vi "main_queque_manager.vi"(8 "error in":errorcluster, 9 "State insert position":T1, 10 "New states array":T2[](array[typedef]), 11 "Main state queue in":refnum<queue>) -> (0 "error out":errorcluster, 3 "Main state queue out":refnum<queue>)   [LabVIEW 2011, in "Fiberscope_library.lvlib"]
uses:
  Fiberscope_library.lvlib
  typedefs/main_state_cluster.ctl
  typedefs/main_state_enum.ctl
  typedefs/state_insert_position_enum.ctl
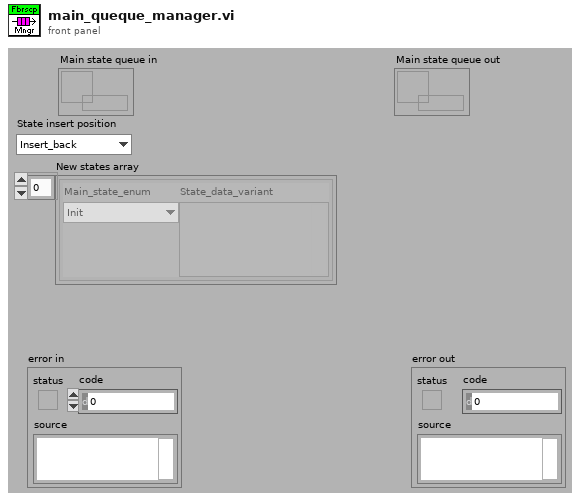
[diagram p1: front panel]
types:
  T1 = typedef "Fiberscope_library.lvlib/state_insert_position_enum.ctl" = enum16{"Insert_back", "Insert_front"}
  T2 = typedef "Fiberscope_library.lvlib/main_state_cluster.ctl" = cluster{"Main_state_enum":T3, "State_data_variant":variant}
  T3 = typedef "Fiberscope_library.lvlib/main_state_enum.ctl" = enum16{"Init", "Error", "Quit", "Run", "Stop", "Parameters_changed", "Timeout", "Pockels", "Shutter"}
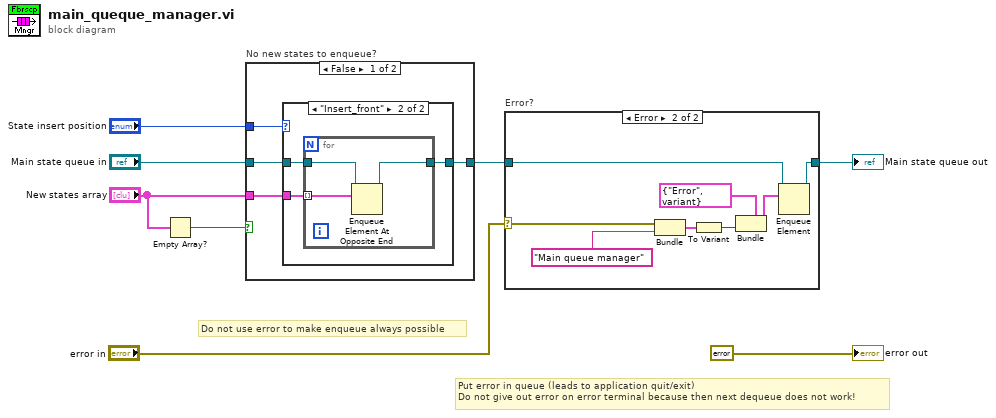
[diagram p0: block diagram]
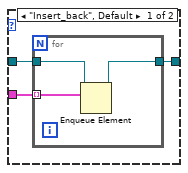
[diagram p3: hidden frame]
diagram:
  # "Put error in queue (leads to application quit/exit)\nDo not give out error on error terminal because then next dequeue does not work!"
  # "Do not use error to make enqueue always possible"
  n1 = Empty Array?(array="New states array") -> (empty?=w8:bool)
  n2 = case "No new states to enqueue?" shown="False" w8 {
    tunnel: "Main state queue in" -> [w11 w25]
    tunnel: [w10 w25] -> w4
    tunnel: "New states array" -> [w12 _]
    tunnel: "State insert position" -> [w9 _]
    frame False {
      n3 = case shown="\"Insert_front\"" w9 {
        tunnel: w12 -> [w15 w19]
        tunnel: w11 -> [w14 w21]
        tunnel: [w13 w20] -> w10
        frame "Insert_back", Default {
          n4 = for {
            tunnel: w15 -> [w18] mode=indexing
            tunnel: w14 -> [w17]
            tunnel: [w16] -> w13
            n5 = Enqueue Element(queue=w17, element=w18) -> (queue out=w16:refnum<queue>)  [unwired: 2 in, 2 out]
          }
        }
        frame "Insert_front" {
          n6 = for {
            tunnel: w19 -> [w24] mode=indexing
            tunnel: w21 -> [w23]
            tunnel: [w22] -> w20
            n7 = Enqueue Element At Opposite End(queue=w23, element=w24) -> (queue out=w22:refnum<queue>)  [unwired: 2 in, 2 out]
          }
        }
      }
    }
    frame True {
    }
  }
  n8 = case "Error?" shown="Error" "error in" {
    selector: "error in" -> [_ w29]
    tunnel: w4 -> [w26 w34]
    tunnel: [w26 w33] -> w3
    frame No Error {
    }
    frame Error {
      n9 = Bundle("error IO"=w29, "Main queue manager") -> (w28:cluster{"error IO":errorcluster, string})  [unwired: 1 in]
      n10 = To Variant(anything=w28) -> (Variant=w32:variant)
      n11 = Bundle(cluster=T2 {"Main_state_enum"=enum."Error", "State_data_variant"=variant} ("Main_state_cluster"), "State_data_variant"=w32) -> (w30:T2)  [unwired: 1 in]
      n12 = Enqueue Element(queue=w34, element=w30) -> (queue out=w33:refnum<queue>)  [unwired: 2 in, 2 out]
    }
  }
  "Main state queue out" <- w3
  "error out" <- errorcluster {"status"=FALSE, "code"=0, "source"=""} ("error out")
